vi "zadanie2.vi"() -> ()   [LabVIEW 2019]
panel:
  in  "Input":string="a"
  in  "String/Int                   Counter":bool=TRUE
  in  "Time Delay for counter":dbl(knob) scale=0.0..1.0
  in  "?":bool
  out "Leds (light = 1)":bool[](array[boolean])
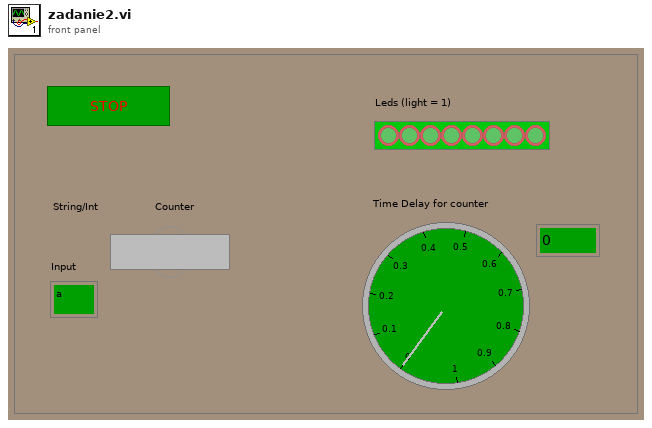
[diagram p1: front panel]
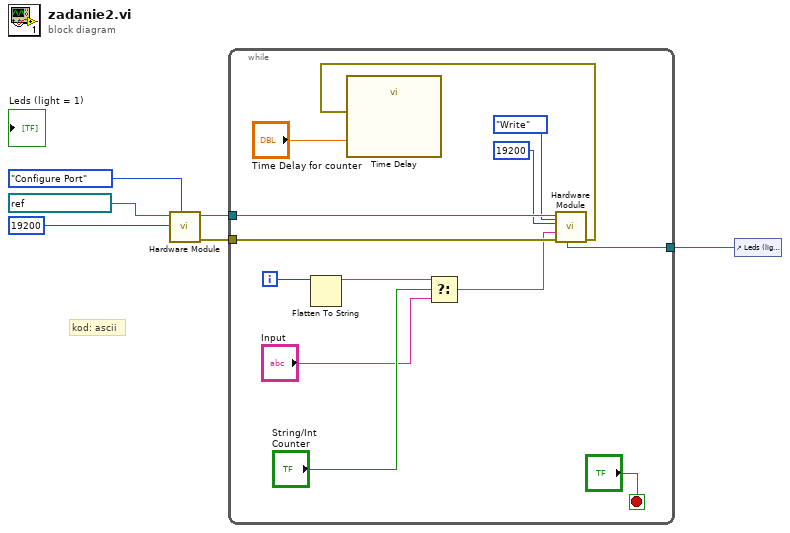
[diagram p0: block diagram]
diagram:
  # "kod: ascii"
  n1 = call "Hardware Module.vi"("State"=enum16{"Configure Port", "Write", "Close"}."Configure Port", "baud rate (9600)"=u32 19200, "VISA resource name"=refnum<visa-resource-name> "VirtualDevice1") -> ("error out"=w6:errorcluster, "VISA resource name out"=w5:refnum<visa-resource-name>)  [unwired: 6 in, 1 out]
  n2 = control-ref of="Leds (light = 1)"() -> (w1:refnum<vi>)
  n3 = while {
    tunnel: w6 -> [w19]
    tunnel: w5 -> [w18]
    tunnel: w1 -> [w15]
    i -> [w8]
    stop <- "?" stop-if-true
    n4 = Flatten To String(anything=w8) -> (data string=w13:string)  [unwired: 3 in, 2 out]
    n5 = Select(t=w13, s="String/Int                   Counter", f="Input") -> (s? t:f=w12:string)
    n6 = call "Hardware Module.vi"("LEDs"=w15, "State"=enum16{"Configure Port", "Write", "Close"}."Write", "error in (no error)"=w19, "write buffer"=w12, "baud rate (9600)"=u32 19200, "VISA resource name"=w18) -> ("error out"=w9:errorcluster)  [unwired: 3 in, 2 out]
    n7 = call "Time Delay"("error in (no error)"=w9, "Delay Time (s)"="Time Delay for counter") -> ()  [unwired: 9 in, 1 out]
  }
